vi "Poly_WriteCOMOut.vi"   [LabVIEW 2012]
doc: "Writes the value of \"Variable In\" to the specified COM \"Port\"."
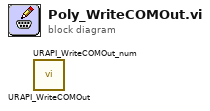
[diagram p0: block diagram]
diagram:
  n1 = call <userlib>:"URAPI_WriteCOMOut.vi"() -> ()  [unwired: 4 in, 2 out]
  n2 = call <userlib>:"URAPI_WriteCOMOut_num.vi"() -> ()  [unwired: 4 in, 2 out]
